vi "sub_strain-cal_onepoint.vi"(11 "strain":dbl) -> (3 "g force":dbl)   [LabVIEW 2016]
uses:
  Global.vi
panel:
  out "XY 그래프":cluster{"X":dbl, "Y":dbl}[](graph)
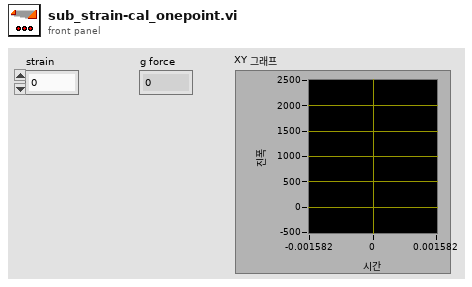
[diagram p1: front panel]
types:
  T1 = typedef "force_sensor_data.ctl" = cluster{"weight":cluster{"front":dbl, "left":dbl, "back":dbl, "right":dbl}, "strain map":cluster{"x":dbl, "y":dbl}[]}
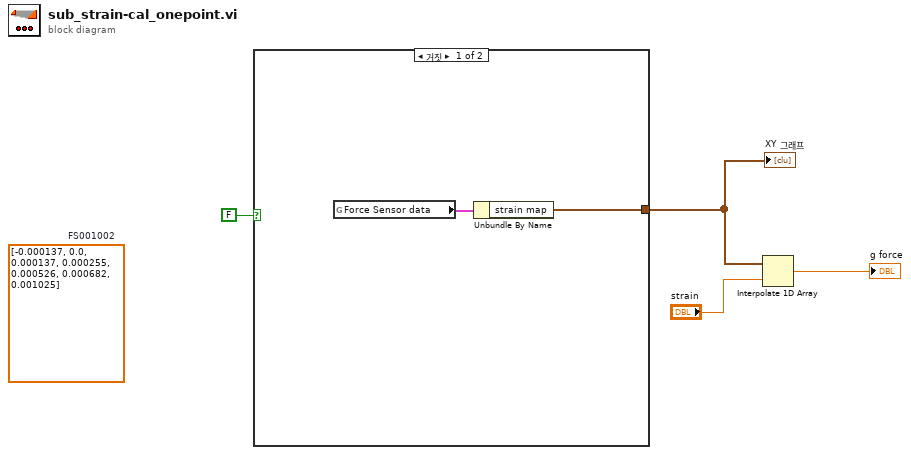
[diagram p0: block diagram]
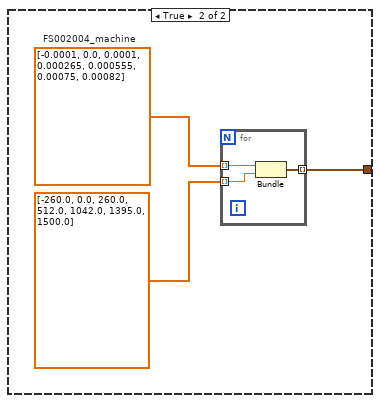
[diagram p2: hidden frame]
diagram:
  (unwired) dbl[] [-0.000137, 0.0, 0.000137, 0.000255, 0.000526, 0.000682, 0.001025]  # FS001002
  n1 = case shown="거짓" FALSE {
    tunnel: [w5 w7] -> w2
    frame False {
      n2 = global read "Global.vi" "Force Sensor data"() -> (w6:T1)
      n3 = Unbundle By Name(w6) -> ("strain map"=w5:cluster{"x":dbl, "y":dbl}[])
    }
    frame True {
      w8 = dbl[] [-0.0001, 0.0, 0.0001, 0.000265, 0.000555, 0.00075, 0.00082]  # FS002004_machine
      n4 = for {
        tunnel: w8 -> [w12] mode=indexing
        tunnel: dbl[] [-260.0, 0.0, 260.0, 512.0, 1042.0, 1395.0, 1500.0] ("y") -> [w11] mode=indexing
        tunnel: [w10] -> w7 mode=indexing
        n5 = Bundle(w12, w11) -> (w10:cluster{dbl, dbl})  [unwired: 1 in]
      }
    }
  }
  "XY 그래프" <- w2
  n6 = Interpolate 1D Array(1:"strain", 2:w2) -> (0:→"g force":dbl)
